vi "dfd_Get Filter Frequency Response.vi"(4 "phase view":T1, 6 "fs [Hz]":dbl=1.0, 7 "# freq bins":i32=512, 8 "error in (no error)":errorcluster, 9 "magnitude":u16(ring) items=["Linear", "dB", "Zero phase"], 10 "coef source":enum16{"Original", "Current", "Quantized"}(ring)=enum."Current", 11 "filter in":T2={"mSRate_Fs"=1.0, "mSRate_Version"="1.0", "mSRate_Comments"="", "mSRate_OrgCoef"={"type"=enum."Undefined", "gain"=1.0, "coef a (k)"=[], "coef b (v)"=[]}, "mSRate_CurCoef"={"type"=enum."Undefined", "gain"=1.0, "coef a (k)"=[], "coef b (v)"=[]}, "mSRate_Quantized?"=FALSE, "mSRate_QCoef"={"type"=enum."Undefined", "gain"=1.0, "coef a (k)"=[], "coef b (v)"=[]}, "mSRate_QSettings"=[], "mSRate_Order"=0, "mSRate_Scaling"={"mSRate_ScaleByPowerOf2?"=FALSE, "mSRate_ScaleType"=enum."No Norm"}} {"mSRate_QSettings"."source" items=["Coef a/k"=0, "Coef b/v"=7, "Input"=1, "Output"=2, "Multiplicand"=3, "Product"=4, "Sum"=5, "Delay"=6, "Gain"=8]}) -> (0 "error out":errorcluster, 1 "df":dbl, 2 "phase":dbl[](array[numeric]), 3 "magnitude":dbl[](array[numeric]), 5 "X(w)":cdb[](array[numeric]))   [LabVIEW 2017, in "NI_DigFilterLicensed.lvlib"]
uses:
  <vilib>/addons/Digital Filter Design/NI_DigFilterLicensed.lvlib
  <vilib>/addons/Digital Filter Design/_Objects.llb/DFD Filter Obj.ctl
  <vilib>/addons/Digital Filter Design/_Objects.llb/DFD Filter Coef.ctl
  <vilib>/addons/Digital Filter Design/_Objects.llb/DFD Filter Structure Type Selector.ctl
  <vilib>/addons/Digital Filter Design/_Objects.llb/dfd_Internal Quantization Settings.ctl
  <vilib>/addons/Digital Filter Design/_Objects.llb/dfd_Internal Quantization Srcs.ctl
  <vilib>/addons/Digital Filter Design/_Objects.llb/DFD Coef Norm Type.ctl
  <vilib>/addons/Digital Filter Design/_Objects.llb/DFD Phase Setting.ctl
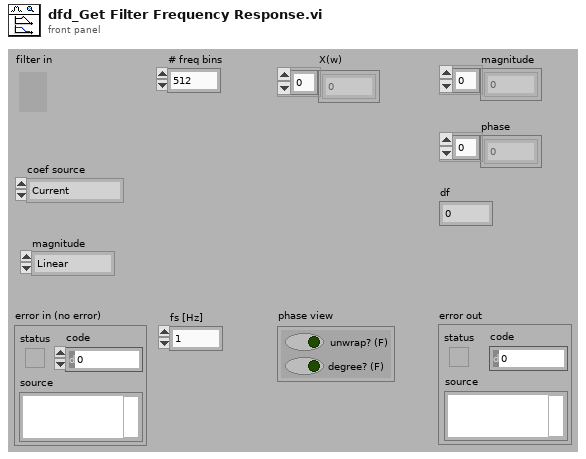
[diagram p1: front panel]
types:
  T1 = typedef "NI_DigFilterLicensed.lvlib/DFD Phase Setting.ctl" = cluster{"unwrap? (F)":bool, "degree? (F)":bool}
  T2 = typedef "NI_DigFilterLicensed.lvlib/DFD Filter Obj.ctl" = cluster{"mSRate_Fs":dbl, "mSRate_Version":string, "mSRate_Comments":string, "mSRate_OrgCoef":T3, "mSRate_CurCoef":T3, "mSRate_Quantized?":bool, "mSRate_QCoef":T3, "mSRate_QSettings":T5[], "mSRate_Order":i32, "mSRate_Scaling":cluster{"mSRate_ScaleByPowerOf2?":bool, "mSRate_ScaleType":T7}}
  T3 = typedef "NI_DigFilterLicensed.lvlib/DFD Filter Coef.ctl" = cluster{"type":T4, "gain":dbl, "coef a (k)":dbl[], "coef b (v)":dbl[]}
  T4 = typedef "NI_DigFilterLicensed.lvlib/DFD Filter Structure Type Selector.ctl" = enum16{"Undefined", "FIR Direct Form", "FIR Direct Form Transposed", "FIR Symmetric", "FIR Antisymmetric", "IIR Direct Form I", "IIR Direct Form I Transposed", "IIR Direct Form II", "IIR Direct Form II Transposed", "IIR Cascaded Second Order Sections Form I", "IIR Cascaded Second Order Sections Form I Transposed", "IIR Cascaded Second Order Sections Form II", "IIR Cascaded Second Order Sections Form II Transposed", "Lattice Allpass (basic sections)", "Lattice Allpass (one multiplier sections)", "Lattice Allpass (normalized sections)", "Lattice AR (basic sections)", "Lattice AR (one multiplier sections)", "Lattice AR (normalized sections)", "Lattice MA (minimum phase)", "Lattice MA (maximum phase)", "Lattice ARMA (basic sections)", "Lattice ARMA (one multiplier sections)", "Lattice ARMA (normalized sections)"}
  T5 = typedef "NI_DigFilterLicensed.lvlib/dfd_Internal Quantization Settings.ctl" = cluster{"source":T6, "wl":i16, "iwl":i16, "overflow mode":enum16{"Saturation", "Wrap"}, "rounding mode":enum16{"Nearest", "Truncation"}, "signed?":bool}
  T6 = typedef "NI_DigFilterLicensed.lvlib/dfd_Internal Quantization Srcs.ctl" = u16
  T7 = typedef "NI_DigFilterLicensed.lvlib/DFD Coef Norm Type.ctl" = enum16{"No Norm", "Time Domain 1-Norm", "Time Domain 2-Norm", "Time Domain Inf-Norm"}
  T8 = typedef "NI_DigFilterLicensed.lvlib/DFD Filter Structure Id.ctl" = enum16{"Undefined", "FIR", "IIR Direct", "IIR SOS", "IIR Allpass", "IIR AR", "IIR ARMA"}
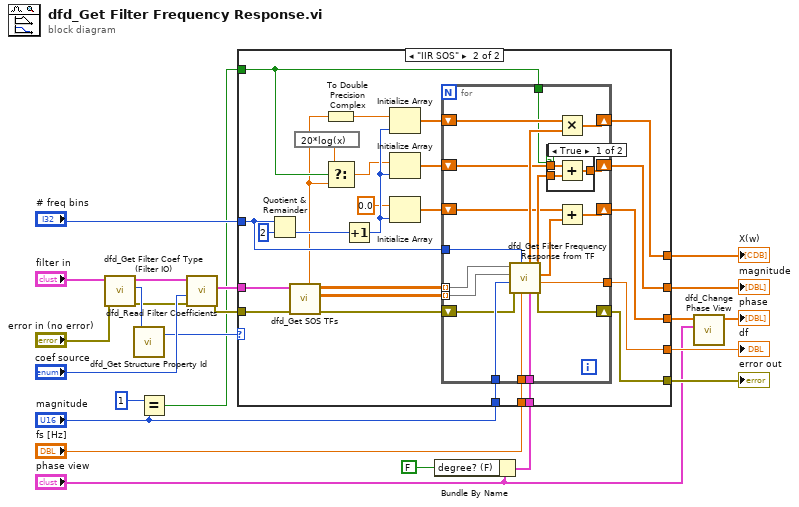
[diagram p0: block diagram]
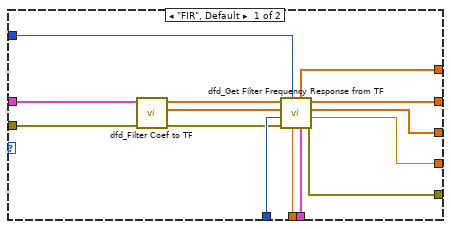
[diagram p2: hidden frame]
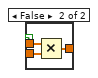
[diagram p3: hidden frame]
diagram:
  n1 = call <vilib>:"dfd_Get Filter Coef Type (Filter IO).vi"("error in (no error)"="error in (no error)", "filter in"="filter in") -> ("error out"=w13:errorcluster, "type"=w14:T4, "filter out"=w11:T2)  [unwired: 1 in, 6 out]
  n2 = call <vilib>:"dfd_Get Structure Property Id.vi"("structure type"=w14) -> ("filter structure id"=w12:T8)  [unwired: 1 out]
  n3 = Equal?(x=u16 1, y="magnitude") -> (x = y?=w9:bool)
  n4 = call <vilib>:"dfd_Read Filter Coefficients.vi"("error in (no error)"=w13, "coef source"="coef source", "filter in"=w11) -> ("error out"=w21:errorcluster, "filter coef"=w19:T3)  [unwired: 7 out]
  n5 = Bundle By Name(cluster="phase view", "degree? (F)"=FALSE) -> (w1:T1)
  n6 = case shown="\"IIR SOS\"" w12 {
    tunnel: [w37 w53] -> w23
    tunnel: [w36 w52] -> w5
    tunnel: [w35 w51] -> w6
    tunnel: "magnitude" -> [w34 w58]
    tunnel: "# freq bins" -> [w33 w57]
    tunnel: w21 -> [w29 w43]
    tunnel: w19 -> [w28 w44]
    tunnel: w1 -> [w27 w55]
    tunnel: [w26 w50] -> w8
    tunnel: "fs [Hz]" -> [w25 w56]
    tunnel: [w24 w38] -> w17
    tunnel: w9 -> [_ w45]
    frame "FIR", Default {
      n7 = call <vilib>:"dfd_Filter Coef to TF.vi"("error out"=w29, "filter coef"=w28) -> ("error"=w32:errorcluster, "denominator"=w31:dbl[], "numerator"=w30:dbl[])  [unwired: 7 out]
      n8 = call <vilib>:"dfd_Get Filter Frequency Response from TF.vi"("phase view"=w27, "fs [Hz]"=w25, "# freq bins (512)"=w33, "error in (no error)"=w32, "magnitude"=w34, "den"=w31, "num"=w30) -> ("error out"=w24:errorcluster, "df"=w37:dbl, "phase"=w36:dbl[], "magnitude"=w35:dbl[], "X(w)"=w26:cdb[])
    }
    frame "IIR SOS" {
      n9 = Quotient & Remainder(x=w57, y=2) -> (floor(x/y)=w62:i32)  [unwired: 1 out]
      n10 = call <vilib>:"dfd_Get SOS TFs.vi"("error in (no error)"=w43, "filter coef"=w44) -> ("error out"=w39:errorcluster, "dens"=w40:dbl[][], "nums"=w41:dbl[][], "gain"=w42:dbl)  [unwired: 6 out]
      n11 = expression code="20*log(x)"(w42) -> (w47:dbl)
      n12 = To Double Precision Complex(1:w42) -> (0:w54:cdb)
      n13 = Select(t=w47, s=w45, f=w42) -> (s? t:f=w46:dbl)
      n14 = Increment(x=w62) -> (x+1=w49:i32)
      n15 = Initialize Array(w54, w49) -> (w61:cdb[])
      n16 = Initialize Array(w46, w49) -> (w60:dbl[])
      n17 = Initialize Array(0.0 ("element"), w49) -> (w59:dbl[])
      n18 = for {
        shift-right: [w74] -> w50
        shift-left: w61 -> [w78]
        shift-right: [w69] -> w51
        shift-left: w60 -> [w76]
        shift-right: [w71] -> w52
        shift-left: w59 -> [w73]
        tunnel: w58 -> [w82]
        tunnel: w57 -> [w81]
        tunnel: w56 -> [w80]
        tunnel: w55 -> [w79]
        tunnel: [w70] -> w53
        tunnel: w45 -> [w68]
        tunnel: w41 -> [w67] mode=indexing
        tunnel: w40 -> [w66] mode=indexing
        shift-right: [w64] -> w38
        shift-left: w39 -> [w65]
        n19 = call <vilib>:"dfd_Get Filter Frequency Response from TF.vi"("phase view"=w79, "fs [Hz]"=w80, "# freq bins (512)"=w81, "error in (no error)"=w65, "magnitude"=w82, "den"=w66, "num"=w67) -> ("error out"=w64:errorcluster, "df"=w70:dbl, "phase"=w72:dbl[], "magnitude"=w75:dbl[], "X(w)"=w77:cdb[])
        n20 = case shown="True" w68 {
          tunnel: w76 -> [w85 w88]
          tunnel: w75 -> [w84 w87]
          tunnel: [w83 w86] -> w69
          frame True {
            n21 = Add(x=w85, y=w84) -> (x+y=w83:dbl[])
          }
          frame False {
            n22 = Multiply(x=w88, y=w87) -> (x*y=w86:dbl[])
          }
        }
        n23 = Multiply(x=w78, y=w77) -> (x*y=w74:cdb[])
        n24 = Add(x=w73, y=w72) -> (x+y=w71:dbl[])
      }
    }
  }
  "df" <- w23
  "error out" <- w17
  "magnitude" <- w6
  "X(w)" <- w8
  n25 = call <vilib>:"dfd_Change Phase View.vi"("phase view"="phase view", "phase in (rad)"=w5) -> ("phase out"=→"phase":dbl[])  [unwired: 9 out]
